vi "Stop Measurements Command.vi"(8 "error in (no error)":errorcluster, 10 "Measurement Controller":string, 11 "Monitor-Pulse in":refnum<class "Batch Processor.lvclass">) -> (0 "error out":errorcluster, 3 "Monitor-Pulse out":refnum<class "Batch Processor.lvclass">)   [LabVIEW 2016, in "Batch Processor.lvclass"]
uses:
  Batch Processor.lvclass
  C:/github/LabActor/Worker/Worker.lvclass
  Worker/Worker State.ctl
  Worker/Worker.lvclass/Worker.ctl
  Template Module/Write State.vi
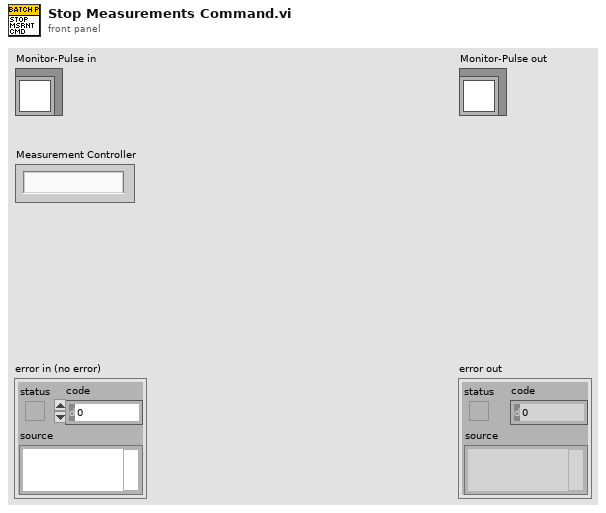
[diagram p1: front panel]
types:
  T1 = typedef "Worker State.ctl" = enum16{"Idle", "Starting", "Working", "Stopping"}
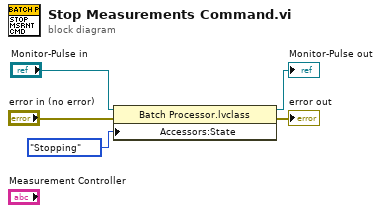
[diagram p0: block diagram]
diagram:
  n1 = property class="Batch Processor.lvclass"(reference="Monitor-Pulse in", error in="error in (no error)", "Accessors:State"=Worker_State."Stopping" ("State")) -> (reference out=→"Monitor-Pulse out":refnum<class "Batch Processor.lvclass">, error out=→"error out":errorcluster)
